vi "Open.vi"(8 "error in (no error)":errorcluster, 11 "TcpSocket in":refnum<class "TcpSocket.lvclass">) -> (0 "error out":errorcluster, 3 "TcpSocket out":refnum<class "TcpSocket.lvclass">)   [LabVIEW 2021, in "TcpSocket.lvlib" / "TcpSocket.lvclass"]
uses:
  TcpSocket.lvclass
  TcpSocket.lvclass/TcpSocket.ctl
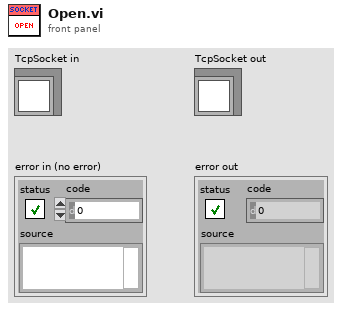
[diagram p1: front panel]
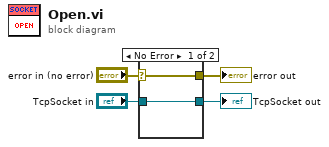
[diagram p0: block diagram]
diagram:
  n1 = case shown="No Error" "error in (no error)" {
    selector: "error in (no error)" -> [w5 w8]
    tunnel: [w5 w8] -> w3
    tunnel: [w6 w7] -> w1
    tunnel: "TcpSocket in" -> [w6 w7]
    frame No Error {
    }
    frame Error {
    }
  }
  "error out" <- w3
  "TcpSocket out" <- w1
